vi "NewVisaRead.vi"(8 "error in (no error)":errorcluster, 11 "VISA Refnum in":refnum<visa-resource-name>) -> (0 "error out":errorcluster, 2 "String":string, 3 "VISA Refnum out":refnum<visa-resource-name>)   [LabVIEW 2020]
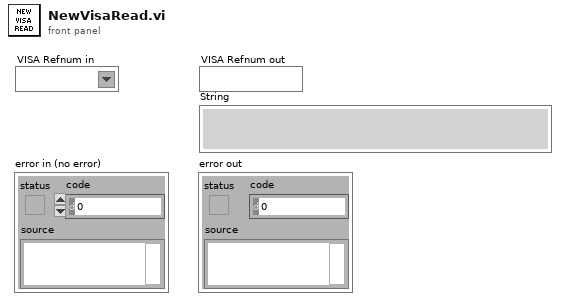
[diagram p1: front panel]
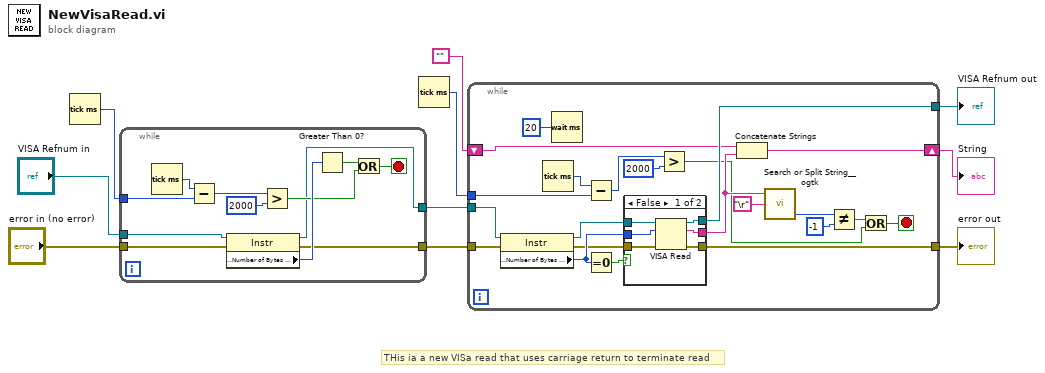
[diagram p0: block diagram]
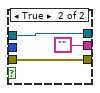
[diagram p2: hidden frame]
diagram:
  # "THis ia a new VISa read that uses carriage return to terminate read"
  n1 = Tick Count (ms)() -> (millisecond timer value=w7:u32)
  n2 = while {
    tunnel: "VISA Refnum in" -> [w22]
    tunnel: w7 -> [w20]
    tunnel: [w15] -> w3
    tunnel: "error in (no error)" -> [w14]
    tunnel: [w13] -> w6
    stop <- w16 stop-if-true
    n3 = Tick Count (ms)() -> (millisecond timer value=w12:u32)
    n4 = Subtract(x=w12, y=w20) -> (x-y=w19:u32)
    n5 = property class="Instr"(reference=w22, error in=w14) -> (reference out=w15:refnum<visa-resource-name>, error out=w13:errorcluster, "Serial Settings:Number of Bytes at Serial Port"=w21:u32)
    n6 = Greater?(x=w19, y=u32 2000) -> (0:w18:bool)
    n7 = Greater Than 0?(x=w21) -> (x > 0?=w17:bool)
    n8 = Or(x=w17, y=w18) -> (x .or. y?=w16:bool)
  }
  n9 = Tick Count (ms)() -> (millisecond timer value=w1:u32)
  n10 = while {
    tunnel: w3 -> [w39]
    tunnel: [w44] -> w9
    shift-right: [w42] -> w10
    shift-left: "" -> [w43]
    tunnel: w6 -> [w40]
    tunnel: [w36] -> w8
    tunnel: w1 -> [w33]
    stop <- w24 stop-if-true
    n11 = property class="Instr"(reference=w39, error in=w40) -> (reference out=w38:refnum<visa-resource-name>, error out=w37:errorcluster, "Serial Settings:Number of Bytes at Serial Port"=w41:u32)
    n12 = Tick Count (ms)() -> (millisecond timer value=w32:u32)
    n13 = Wait (ms)(milliseconds to wait=u32 20) -> ()  [unwired: 1 out]
    n14 = Subtract(x=w32, y=w33) -> (x-y=w34:u32)
    n15 = Equal To 0?(x=w41) -> (x = 0?=w30:bool)
    n16 = case shown="False" w30 {
      tunnel: w38 -> [w50 w52]
      tunnel: [w49 w52] -> w44
      tunnel: [w48 ""] -> w29
      tunnel: w41 -> [w47 _]
      tunnel: w37 -> [w46 w51]
      tunnel: [w45 w51] -> w36
      frame False {
        n17 = VISA Read(VISA resource name=w50, byte count=w47, error in (no error)=w46) -> (VISA resource name out=w49:refnum<visa-resource-name>, read buffer=w48:string, error out=w45:errorcluster)  [unwired: 1 out]
      }
      frame True {
      }
    }
    n18 = Greater?(x=w34, y=u32 2000) -> (0:w23:bool)
    n19 = Concatenate Strings(w43, w29) -> (w42:string)
    n20 = call "Search or Split String__ogtk.vi"("search string/char (-)"="\r", "string"=w29) -> ("offset after match"=w27:i32)  [unwired: 1 in, 2 out]
    n21 = Not Equal?(x=w27, y=-1) -> (x != y?=w25:bool)
    n22 = Or(x=w25, y=w23) -> (x .or. y?=w24:bool)
  }
  "String" <- w10
  "VISA Refnum out" <- w9
  "error out" <- w8
